vi "Get File Extension.vi"(8 "error in (no error)":errorcluster, 11 "SPXMusicLibrary in":refnum<class "SPXMusicLibrary.lvclass">) -> (0 "error out":errorcluster, 2 "File Extention":string, 3 "SPXMusicLibrary out":refnum<class "SPXMusicLibrary.lvclass">)   [LabVIEW 2015, in "SPXMusicLibrary.lvclass"]
uses:
  SPXMusicLibrary.lvclass
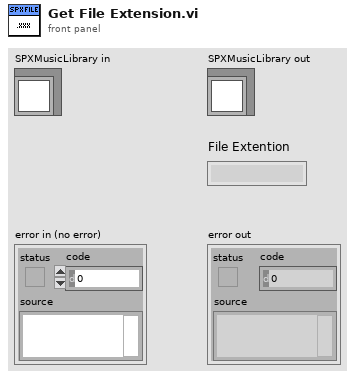
[diagram p1: front panel]
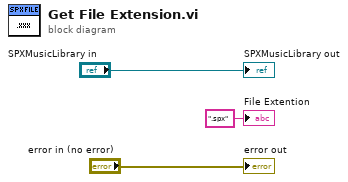
[diagram p0: block diagram]
diagram:
  "error out" <- "error in (no error)"
  "SPXMusicLibrary out" <- "SPXMusicLibrary in"
  "File Extention" <- ".spx" ("File Extention")
